vi "CLD 13 Flow Rates Exercise.vi"() -> ()   [LabVIEW 2014]
doc: "CLD-Übung 13"
uses:
  CLD 13 Data Cluster.ctl
  CLD 13 State Machine Enum.ctl
  CLD 13 timer Enum.ctl
panel:
  out "Fehler (Ausgang)":T1
  in  "Fehler (Eingang)":T1
  out "Durchflussmesser":i8(knob) scale=-20.0..20.0 scale format="%_2f"
  in  "Applikation stoppen":bool
  in  "Durchfluss stoppen":bool
  out "Verstrichene Zeit":dbl
  out "Flussrate":dbl
  in  "Flussratenänderung":i8(slide) min=-2 max=2 step=1 scale=-2.0..2.0
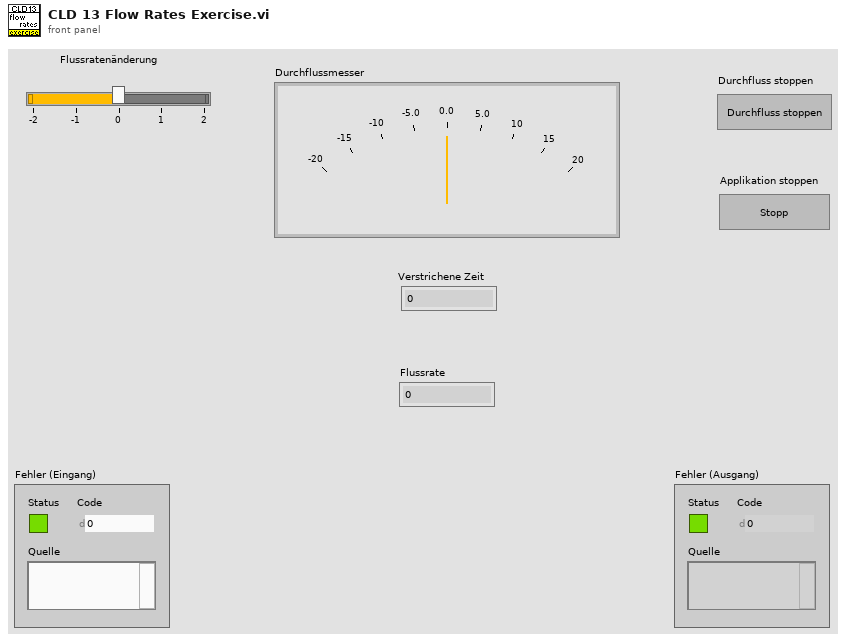
[diagram p1: front panel]
types:
  T1 = cluster{"Status":bool, "Code":i32, "Quelle":string}
  T2 = typedef "CLD 13 timer Enum.ctl" = enum16{"Starten", "Lesen"}
  T3 = typedef "CLD 13 State Machine Enum.ctl" = enum16{"Initialisieren", "Ruhezustand", "Durchfluss stoppen", "Prozess"}
  T4 = typedef "CLD 13 Data Cluster.ctl" = cluster{"Flussratenänderung":i8, "Flussrate":i8}
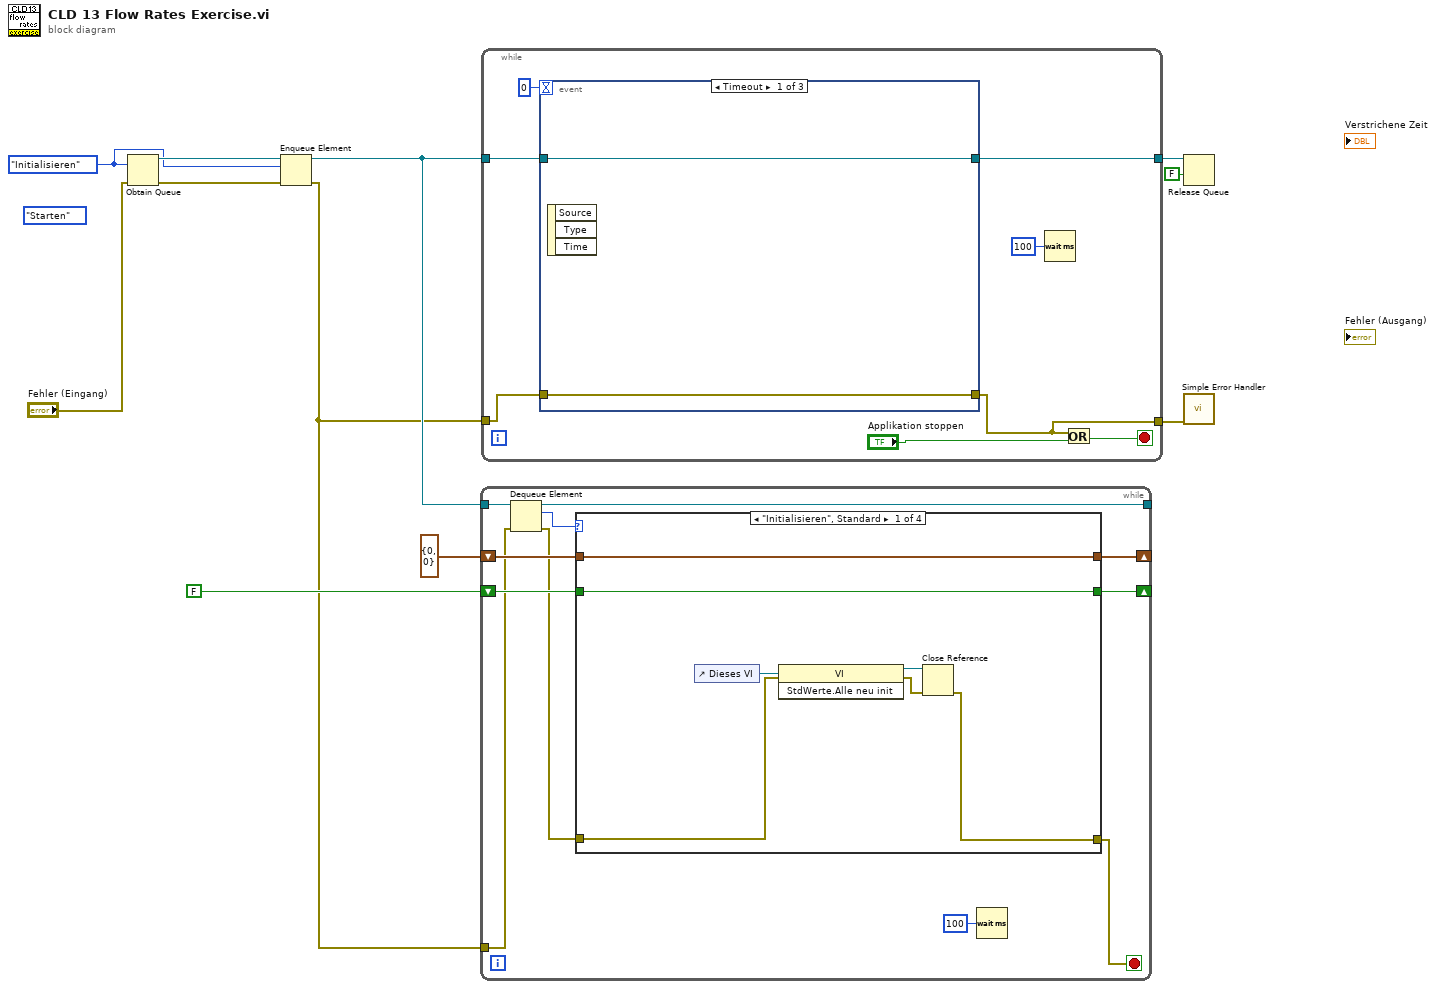
[diagram p0: block diagram]
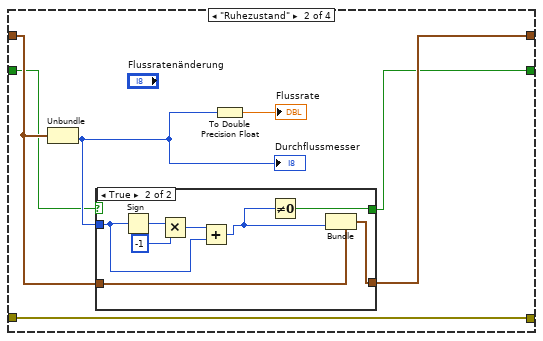
[diagram p2: hidden frame]
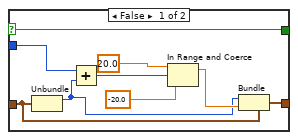
[diagram p3: hidden frame]
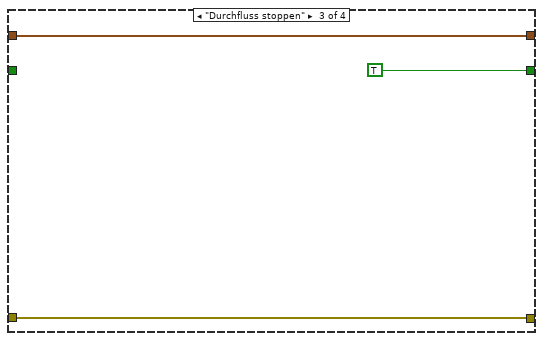
[diagram p4: hidden frame]
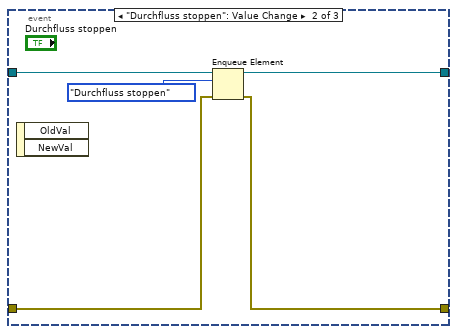
[diagram p6: hidden frame]
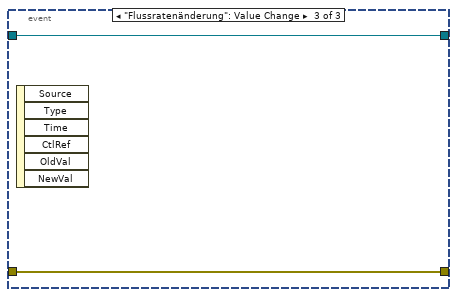
[diagram p7: hidden frame]
diagram:
  (unwired) CLD_13_timer_Enum."Starten" ("Timer-Enum")
  w7 = CLD_13_State_Machine_Enum."Initialisieren" ("CLD 13")
  n1 = Obtain Queue(element data type=w7, error in (no error)="Fehler (Eingang)") -> (queue out=w11:refnum<queue>, error out=w8:errorcluster)  [unwired: 3 in, 1 out]
  n2 = Enqueue Element(queue=w11, element=w7, error in (no error)=w8) -> (queue out=w9:refnum<queue>, error out=w6:errorcluster)  [unwired: 1 in, 1 out]
  n3 = while {
    tunnel: w9 -> [w22]
    tunnel: w6 -> [w13]
    tunnel: [w21] -> _
    shift-right: [w18] -> _
    shift-left: FALSE -> [w19]
    shift-right: [w16] -> _
    shift-left: T4 {"Flussratenänderung"=0, "Flussrate"=0} ("Cluster") -> [w17]
    stop <- w15 stop-if-true
    n4 = Dequeue Element(queue=w22, error in (no error)=w13) -> (queue out=w21:refnum<queue>, element=w20:T3, error out=w14:errorcluster)  [unwired: 1 in, 1 out]
    n5 = case shown="\"Initialisieren\", Standard" w20 {
      tunnel: w19 -> [w29 w32 _ w59]
      tunnel: [w29 w31 TRUE w59] -> w18
      tunnel: w17 -> [w28 w34 w55 w58]
      tunnel: [w28 w33 w55 w58] -> w16
      tunnel: [w24 w30 w54 w57] -> w15
      tunnel: w14 -> [w23 w30 w54 w57]
      frame "Initialisieren", Default {
        n6 = control-ref of="Dieses VI"() -> (w27:refnum<vi>)
        n7 = invoke class="VI" method="StdWerte.Alle neu init"(reference=w27, error in=w23) -> (reference out=w25:refnum<vi>, error out=w26:errorcluster)  [unwired: 1 in, 1 out]
        n8 = Close Reference(reference=w25, error in (no error)=w26) -> (error out=w24:errorcluster)
      }
      frame "Ruhezustand" {
        n9 = Unbundle(w34) -> ("Flussrate"=w35:i8)  [unwired: 1 out]
        "Durchflussmesser" <- w35
        n10 = case shown="True" w32 {
          selector: w32 -> [w37 _]
          tunnel: w35 -> [w45 w48]
          tunnel: w34 -> [w38 w51]
          tunnel: [w41 w50] -> w33
          tunnel: [w37 w46] -> w31
          frame False {
            n11 = Unbundle(w38) -> ("Flussratenänderung"=w39:i8)  [unwired: 1 out]
            n12 = Add(x=w45, y=w39) -> (x+y=w42:i8)
            n13 = In Range and Coerce(upper limit=20.0 ("Obergrenze"), x=w42, lower limit=-20.0 ("Untergrenze")) -> (coerced(x)=w40:dbl)  [unwired: 1 out]
            n14 = Bundle(cluster=w38, "Flussratenänderung"=w39, "Flussrate"=w40) -> (w41:T4)
          }
          frame True {
            n15 = Sign(1:w48) -> (0:w53:i8)
            n16 = Multiply(x=w53, y=i8 -1) -> (x*y=w49:i8)
            n17 = Add(x=w49, y=w48) -> (x+y=w47:i8)
            n18 = Not Equal To 0?(x=w47) -> (x != 0?=w46:bool)
            n19 = Bundle(cluster=w51, "Flussrate"=w47) -> (w50:T4)  [unwired: 1 in]
          }
        }
        n20 = To Double Precision Float(number=w35) -> (double precision float=→"Flussrate":dbl)
      }
      frame "Durchfluss stoppen" {
      }
      frame "Prozess" {
      }
    }
    n21 = Wait (ms)(milliseconds to wait=u32 100 ("Zu wartende ms")) -> ()  [unwired: 1 out]
  }
  n22 = while {
    tunnel: w9 -> [w67]
    tunnel: w6 -> [w64]
    tunnel: [w65] -> w4
    tunnel: [w62] -> w3
    stop <- w63 stop-if-true
    n23 = event shown="[0] Timeout" {
      selector: _ -> [_ _ _]
      dyn-events: _ -> [_ _ _]
      timeout: 0 -> [_ _ _]
      tunnel: w67 -> [w69 w74 w76]
      tunnel: [w69 w73 w76] -> w65
      tunnel: w64 -> [w68 w71 w75]
      tunnel: [w68 w70 w75] -> w62
      event Timeout {
        n24 = event-data() -> ()  [unwired: 1 in, 3 out]
      }
      event "Durchfluss stoppen": Value Change {
        n25 = event-data() -> ()  [unwired: 1 in, 2 out]
        n26 = Enqueue Element(queue=w74, element=CLD_13_State_Machine_Enum."Durchfluss stoppen" ("CLD 13"), error in (no error)=w71) -> (queue out=w73:refnum<queue>, error out=w70:errorcluster)  [unwired: 1 in, 1 out]
      }
      event "Flussratenänderung": Value Change {
        n27 = event-data() -> ()  [unwired: 1 in, 6 out]
      }
    }
    n28 = Wait (ms)(milliseconds to wait=u32 100 ("Zu wartende ms")) -> ()  [unwired: 1 out]
    n29 = Or(x=w62, y="Applikation stoppen") -> (x .or. y?=w63:bool)
  }
  n30 = Release Queue(queue=w4, force destroy? (F)=FALSE ("Eliminieren? (F)")) -> ()  [unwired: 1 in, 3 out]
  n31 = call <vilib>:"Simple Error Handler.vi"("error in (no error)"=w3) -> ()  [unwired: 4 in, 5 out]
